vi "Acqui_temperature.vi"() -> ()   [LabVIEW 2017]
uses:
  <vilib>/DAQmx/read.llb/DAQmx Read (Counter U32 1Chan 1Samp).vi
  <vilib>/DAQmx/create/channels.llb/DAQmx Create Channel (CI-Count Edges).vi
  <vilib>/DAQmx/miscellaneous.llb/DAQmx Fill In Error Info.vi
  <resource>/objmgr/daqmx.rc
panel:
  out "Data":u32 caption="données"
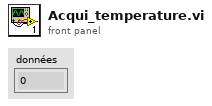
[diagram p1: front panel]
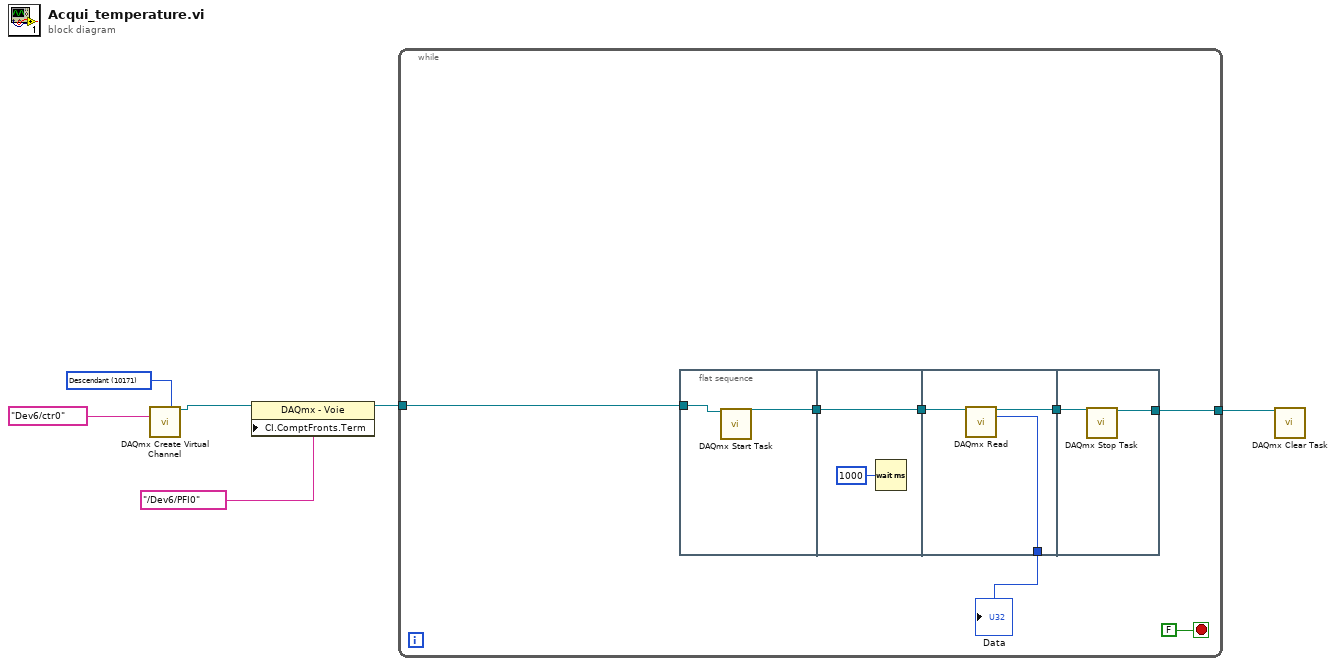
[diagram p0: block diagram]
diagram:
  w4 = 10171 items=["Montant"=10280, "Descendant"=10171] ("edge")
  n1 = call-poly <vilib>:"DAQmx Create Virtual Channel.vi"("edge"=w4, "counter"=tag "Dev6/ctr0") -> ("task out"=w2:refnum<k21>)  [unwired: 12 in, 1 out]
  n2 = property class="DAQmx - Voie"(reference=w2, "CI.ComptFronts.Term"=tag "/Dev6/PFI0") -> (reference out=w5:refnum<k21>)  [unwired: 1 in, 1 out]
  n3 = while {
    tunnel: [w12] -> w6
    tunnel: w5 -> [w7]
    stop <- FALSE stop-if-true
    n4 = flat-sequence {
      tunnel: [w15] -> w9
      tunnel: w7 -> [w14]
      tunnel: w9 -> [w16]
      tunnel: [w16] -> w8
      tunnel: [w20] -> w11
      tunnel: [w19] -> w10
      tunnel: w8 -> [w18]
      tunnel: [w22] -> w12
      tunnel: w11 -> [w21]
      frame #0 {
        n5 = call <vilib>:"DAQmx Start Task.vi"("task/channels in"=w14) -> ("task out"=w15:refnum<k21>)  [unwired: 13 in, 1 out]
      }
      frame #1 {
        n6 = Wait (ms)(milliseconds to wait=u32 1000 ("attente (ms)")) -> ()  [unwired: 1 out]
      }
      frame #2 {
        n7 = call-poly <vilib>:"DAQmx Read.vi"("task/channels in"=w18) -> ("task out"=w20:refnum<k21>, "data"=w19:u32)  [unwired: 12 in, 1 out]
      }
      frame #3 {
        n8 = call <vilib>:"DAQmx Stop Task.vi"("task/channels in"=w21) -> ("task out"=w22:refnum<k21>)  [unwired: 13 in, 1 out]
      }
    }
    "Data" <- w10
  }
  n9 = call <vilib>:"DAQmx Clear Task.vi"("task in"=w6) -> ()  [unwired: 14 in, 1 out]
